vi "Calculate Frequency Error.vi"(11 "Sampling Time":dbl format="%#_13g") -> (3 "df":dbl format="%#_13g")   [LabVIEW 2018]
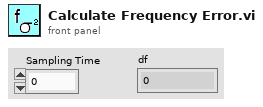
[diagram p1: front panel]
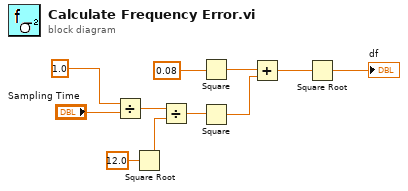
[diagram p0: block diagram]
diagram:
  n1 = Divide(x=1.0, y="Sampling Time") -> (x/y=w2:dbl)
  n2 = Square Root(x=12.0) -> (sqrt(x)=w4:dbl)
  n3 = Divide(x=w2, y=w4) -> (x/y=w5:dbl)
  n4 = Square(x=0.08) -> (x^2=w8:dbl)
  n5 = Square(x=w5) -> (x^2=w7:dbl)
  n6 = Add(x=w8, y=w7) -> (x+y=w11:dbl)
  n7 = Square Root(x=w11) -> (sqrt(x)=→"df":dbl)
